vi "SEE_PXI_TopBench_Rev11.vi"() -> ()   [LabVIEW 2019]
uses:
  Controls/DataBlockControl.ctl
  Controls/RFBlockControl.ctl
  <instrlib>/niScope/Controls/niScope vertical coupling.ctl
  Controls/VISA_power_Control.ctl
  Controls/DCPowerBlock_byInstrument_Control.ctl
  Controls/OscilloscopeBlockControl2.ctl
  Controls/PlotColorArray.ctl
panel:
  in  "output cluster":T6 {"Oscilloscope Configuration Input Array"."vertical coupling" items=["AC", "DC", "Ground"]}
  out "DCPowerInformationArrayOutput":T1[](array[typedef])
  in  "DCPowerInformationClusterArray_Input":T1[](array[typedef])
  in  "config file inputs":T7 {"Oscilloscope Configuration Input Array"."vertical coupling" items=["AC", "DC", "Ground"]}
  out "VISAPowerOutputArray":T2[](array[typedef])
  out "OscilloscopeInfoArray":T8(array[cluster]) {"vertical coupling" items=["AC", "DC", "Ground"]}
  out "RFBlockInfoArray":T3[](array[typedef])
  out "error in":errorcluster
  out "Run Parameters":T9
  in  "stop":bool
  out "Configuration Dashboard":bool[](array[boolean])
  in  "Data Collection Block":bool
  in  "Oscilloscope Block":bool
  in  "Power Block":bool
  in  "RF Block":bool
  in  "Data Block":bool
  in  "Reset":bool
  # "Instructions:\nProgress through the configuration dashboard, note the arrays to the right to confirm settings. Once everything is configured, you can begin data collection"
  # "IMPORTANT NOTES\n\nALL LEDs must be lit up before you can begin data collection. Even if you don't need an RF source or oscilloscope, you still just open up the system and then exit (you don't need to configure one.\n\nAfter data collection, you will have the option to reset the system or keep the configuration.\n\nOnly press \"stop\" if you are completely done with collecting data or if the program does not allow you to open another subvi\n\nIf you get a \"running an implicit call\" just restart the program"
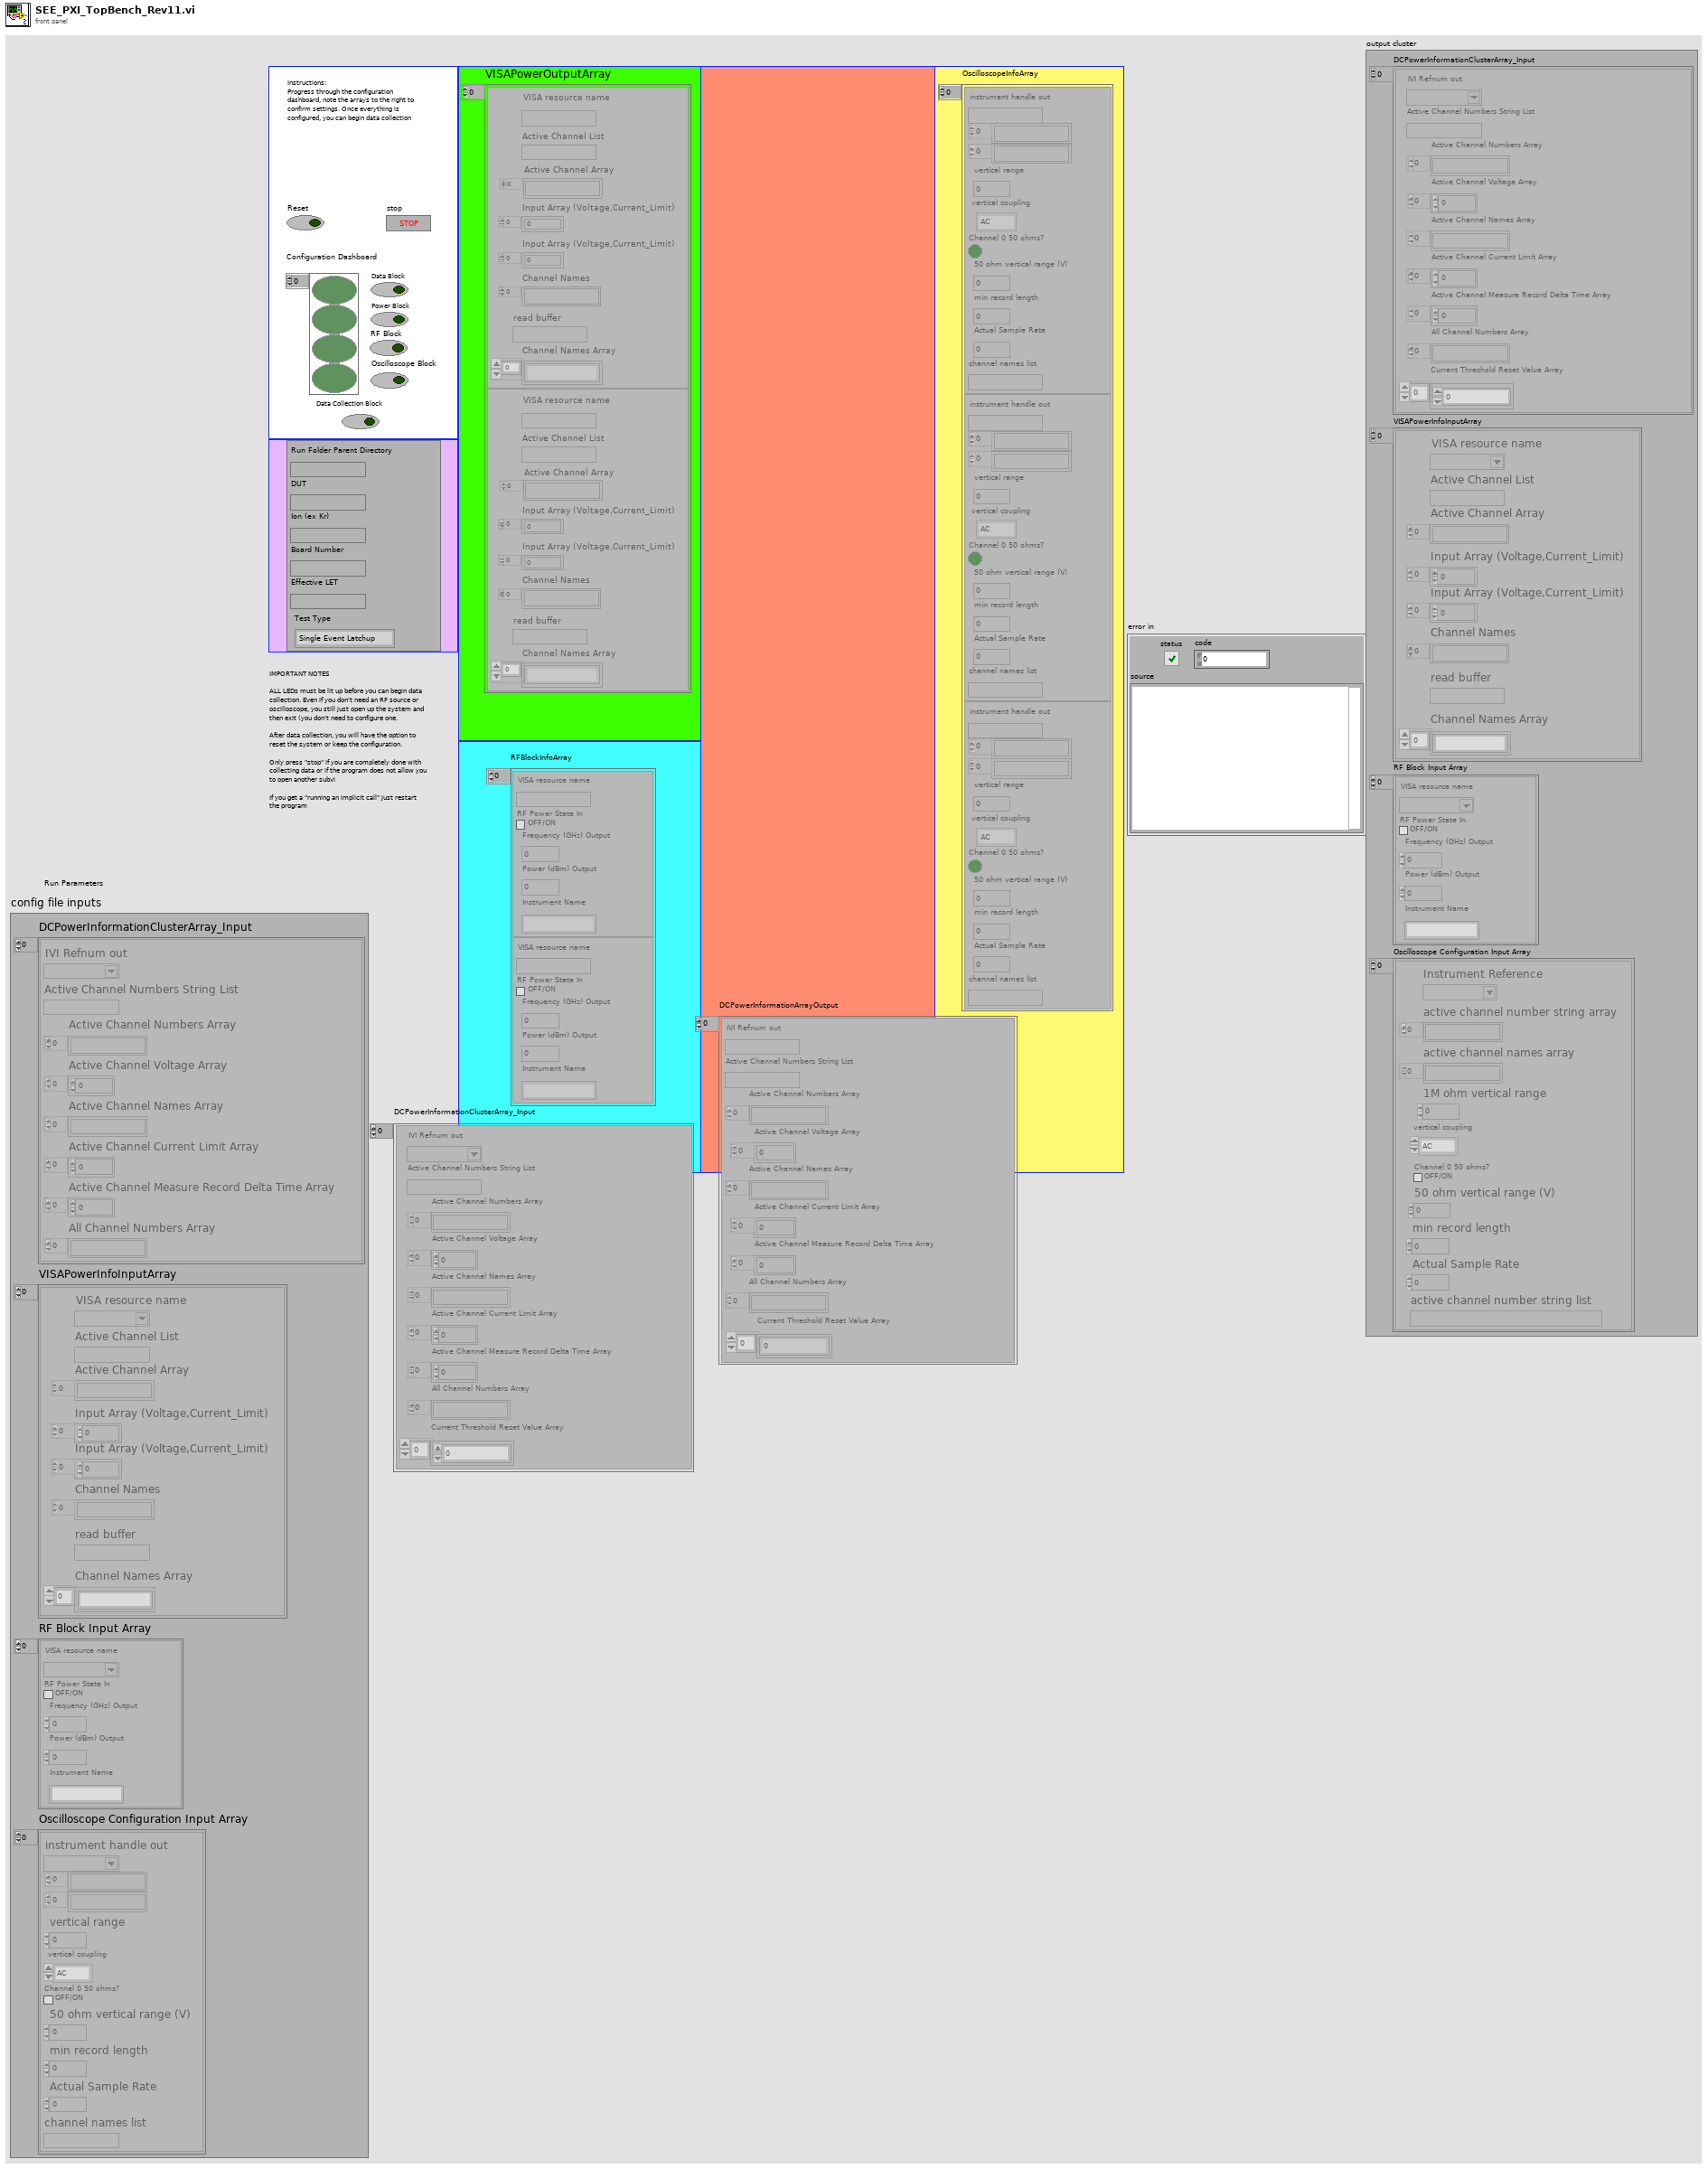
[diagram p1: front panel]
types:
  T1 = typedef "DCPowerBlock_byInstrument_Control.ctl" = cluster{"IVI Refnum out":refnum<k15>, "Active Channel Numbers String List":string, "Active Channel Numbers Array":string[], "Active Channel Voltage Array":dbl[], "Active Channel Names Array":string[], "Active Channel Current Limit Array":dbl[], "Active Channel Measure Record Delta Time Array":dbl[], "All Channel Numbers Array":string[], "Current Threshold Reset Value Array":dbl[]}
  T2 = typedef "VISA_power_Control.ctl" = cluster{"VISA resource name":refnum<visa-resource-name>, "Active Channel List":string, "Active Channel Array":string[], "Input Array (Voltage,Current_Limit)":dbl[], "Input Array (Voltage,Current_Limit)":dbl[], "Channel Names":string[], "read buffer":string, "Channel Names Array":string[]}
  T3 = typedef "RFBlockControl.ctl" = cluster{"VISA resource name":refnum<visa-resource-name>, "RF Power State In":bool, "Frequency (GHz) Output":dbl, "Power (dBm) Output":dbl, "Instrument Name":string}
  T4 = typedef "OscilloscopeBlockControl2.ctl" = cluster{"Instrument Reference":refnum<k15>, "active channel number string array":string[], "active channel names array":string[], "1M ohm vertical range":dbl, "vertical coupling":T5, "Channel 0 50 ohms?":bool, "50 ohm vertical range (V)":dbl, "min record length":i32, "Actual Sample Rate":dbl, "active channel number string list":string}
  T5 = typedef "niScope vertical coupling.ctl" = i32
  T6 = cluster{"DCPowerInformationClusterArray_Input":T1[], "VISAPowerInfoInputArray":T2[], "RF Block Input Array":T3[], "Oscilloscope Configuration Input Array":T4[]}
  T7 = cluster{"DCPowerInformationClusterArray_Input":cluster{"IVI Refnum out":refnum<k15>, "Active Channel Numbers String List":string, "Active Channel Numbers Array":string[], "Active Channel Voltage Array":dbl[], "Active Channel Names Array":string[], "Active Channel Current Limit Array":dbl[], "Active Channel Measure Record Delta Time Array":dbl[], "All Channel Numbers Array":string[]}[], "VISAPowerInfoInputArray":T2[], "RF Block Input Array":T3[], "Oscilloscope Configuration Input Array":cluster{"instrument handle out":refnum<k15>, string[], string[], "vertical range":dbl, "vertical coupling":T5, "Channel 0 50 ohms?":bool, "50 ohm vertical range (V)":dbl, "min record length":i32, "Actual Sample Rate":dbl, "channel names list":string}[]}
  T8 = cluster{"instrument handle out":refnum<k15>, string[], string[], "vertical range":dbl, "vertical coupling":T5, "Channel 0 50 ohms?":bool, "50 ohm vertical range (V)":dbl, "min record length":i32, "Actual Sample Rate":dbl, "channel names list":string}[]
  T9 = typedef "DataBlockControl.ctl" = cluster{"Run Folder Parent Directory":path, "DUT":string, "Ion (ex Kr)":string, "Board Number":string, "Effective LET":string, "Test Type":enum16{"Single Event Latchup", "Single Event Transient", "Single Event Upset"}}
  T10 = cluster{"product_name":string, "register_read_array":dbl[], "performance_check":string, "campaign":string, "logic_path":string, "logic_name":string, "power_supplies":cluster{"Supply_Number":dbl, "Supply_Array":cluster{"instr_name":string, "voltage":dbl, "supply_name":string, "channel":string, "current_limit":dbl, "measure_record_length":dbl, "aperature_time":dbl}[]}, "signal_generators":cluster{"Gen_Number":dbl, "Gen_Array":cluster{"GPIB_address":dbl, "signal_name":string, "frequency":dbl, "power":dbl}[]}, "expected_register_values":cluster{"Reg_0x3":string}}
  T11 = typedef "PlotColorArray.ctl" = u32[]
  T12 = cluster{"instrument handle out":refnum<k15>, string, string[], dbl[], string[], "Current Limit Output Array":dbl[], dbl[]}[]
  T13 = cluster{"DCPowerInformationClusterArray_Input":cluster{"IVI Refnum out":refnum<k15>, "Active Channel Numbers String List":string, "Active Channel Numbers Array":string[], "Active Channel Voltage Array":dbl[], "Active Channel Names Array":string[], "Active Channel Current Limit Array":dbl[], "Active Channel Measure Record Delta Time Array":dbl[], "All Channel Numbers Array":string[]}[], "VISAPowerInfoInputArray":cluster{"VISA resource name":refnum<visa-resource-name>, "String List":string, string[], "Input Array (Voltage,Current_Limit)":dbl[], "Input Array (Voltage,Current_Limit)":dbl[], "Channel Names":string[], "read buffer":string}[], "RF Block Input Array":T3[], "Oscilloscope Configuration Input Array":cluster{"instrument handle out":refnum<k15>, string[], string[], "vertical range":dbl, "vertical coupling":T5, "Channel 0 50 ohms?":bool, "50 ohm vertical range (V)":dbl, "min record length":i32, "Actual Sample Rate":dbl, "channel names list":string}[]}
  T14 = cluster{"VISA resource name":refnum<visa-resource-name>, "String List":string, string[], "Input Array (Voltage,Current_Limit)":dbl[], "Input Array (Voltage,Current_Limit)":dbl[], "Channel Names":string[], "read buffer":string}[]
  T15 = cluster{"IVI Refnum out":refnum<k15>, "Active Channel Numbers String List":string, "Active Channel Numbers Array":string[], "Active Channel Voltage Array":dbl[], "Active Channel Names Array":string[], "Active Channel Current Limit Array":dbl[], "Active Channel Measure Record Delta Time Array":dbl[], "All Channel Numbers Array":string[]}[]
  T16 = cluster{"IVI Refnum out":refnum<k15>, "String List":string, string[], dbl[], string[], dbl[], dbl[], string[], dbl[]}[]
  T17 = cluster{"instrument handle out":refnum<k15>, "channel numbers array":string[], "channel names array":string[], "vertical range":dbl, "vertical coupling":T5, "Channel 0 50 ohms?":bool, "50 ohm vertical range (V)":dbl, "min record length":i32, "Actual Sample Rate":dbl}[]
  T18 = enum16{"Single Event Latchup", "Single Event Transient", "Single Event Upset"}
  T19 = cluster{"Array of fetched data":dbl[][], string, i32[]}[]
  T20 = cluster{"Array of fetched data":dbl[][], string, i32[]}[][]
  T21 = cluster{"Array of fetched data":dbl[][], string, i32[]}
  T22 = cluster{"IVI Refnum out":refnum<k15>, "Active Channel Numbers String List":string, "Active Channel Numbers Array":string[], "Active Channel Voltage Array":dbl[], "Active Channel Names Array":string[], "Active Channel Current Limit Array":dbl[], "Active Channel Measure Record Delta Time Array":dbl[], "All Channel Numbers Array":string[], dbl[]}[]
  T23 = cluster{"DCPowerInformationClusterArray_Input out":cluster{"IVI Refnum out":refnum<k15>, "Active Channel Numbers String List":string, "Active Channel Numbers Array":string[], "Active Channel Voltage Array":dbl[], "Active Channel Names Array":string[], "Active Channel Current Limit Array":dbl[], "Active Channel Measure Record Delta Time Array":dbl[], "All Channel Numbers Array":string[]}[], "VISAPowerInfoInputArray":cluster{"VISA resource name":refnum<visa-resource-name>, "String List":string, string[], "Input Array (Voltage,Current_Limit)":dbl[], "Input Array (Voltage,Current_Limit)":dbl[], "Channel Names":string[], "read buffer":string}[], "RF Block Input Array out":T3[], "Oscilloscope Configuration Input Array":cluster{"instrument handle out":refnum<k15>, string[], string[], "vertical range":dbl, "vertical coupling":T5, "Channel 0 50 ohms?":bool, "50 ohm vertical range (V)":dbl, "min record length":i32, "Actual Sample Rate":dbl, "channel names list":string}[]}
  T24 = cluster{"path out":path, string, "Ion (ex Kr)":string, "Board Number":string, "Effective LET":string, "Test Type":enum16{"Single Event Latchup", "Single Event Transient", "Single Event Upset"}}
  T25 = cluster{"DCPowerInformationClusterArray out":T1[], "VISAPowerInfoOutputArray":T2[], "RF Block Input Array out":T3[], "Oscilloscope Configuration Input Array":T4[]}
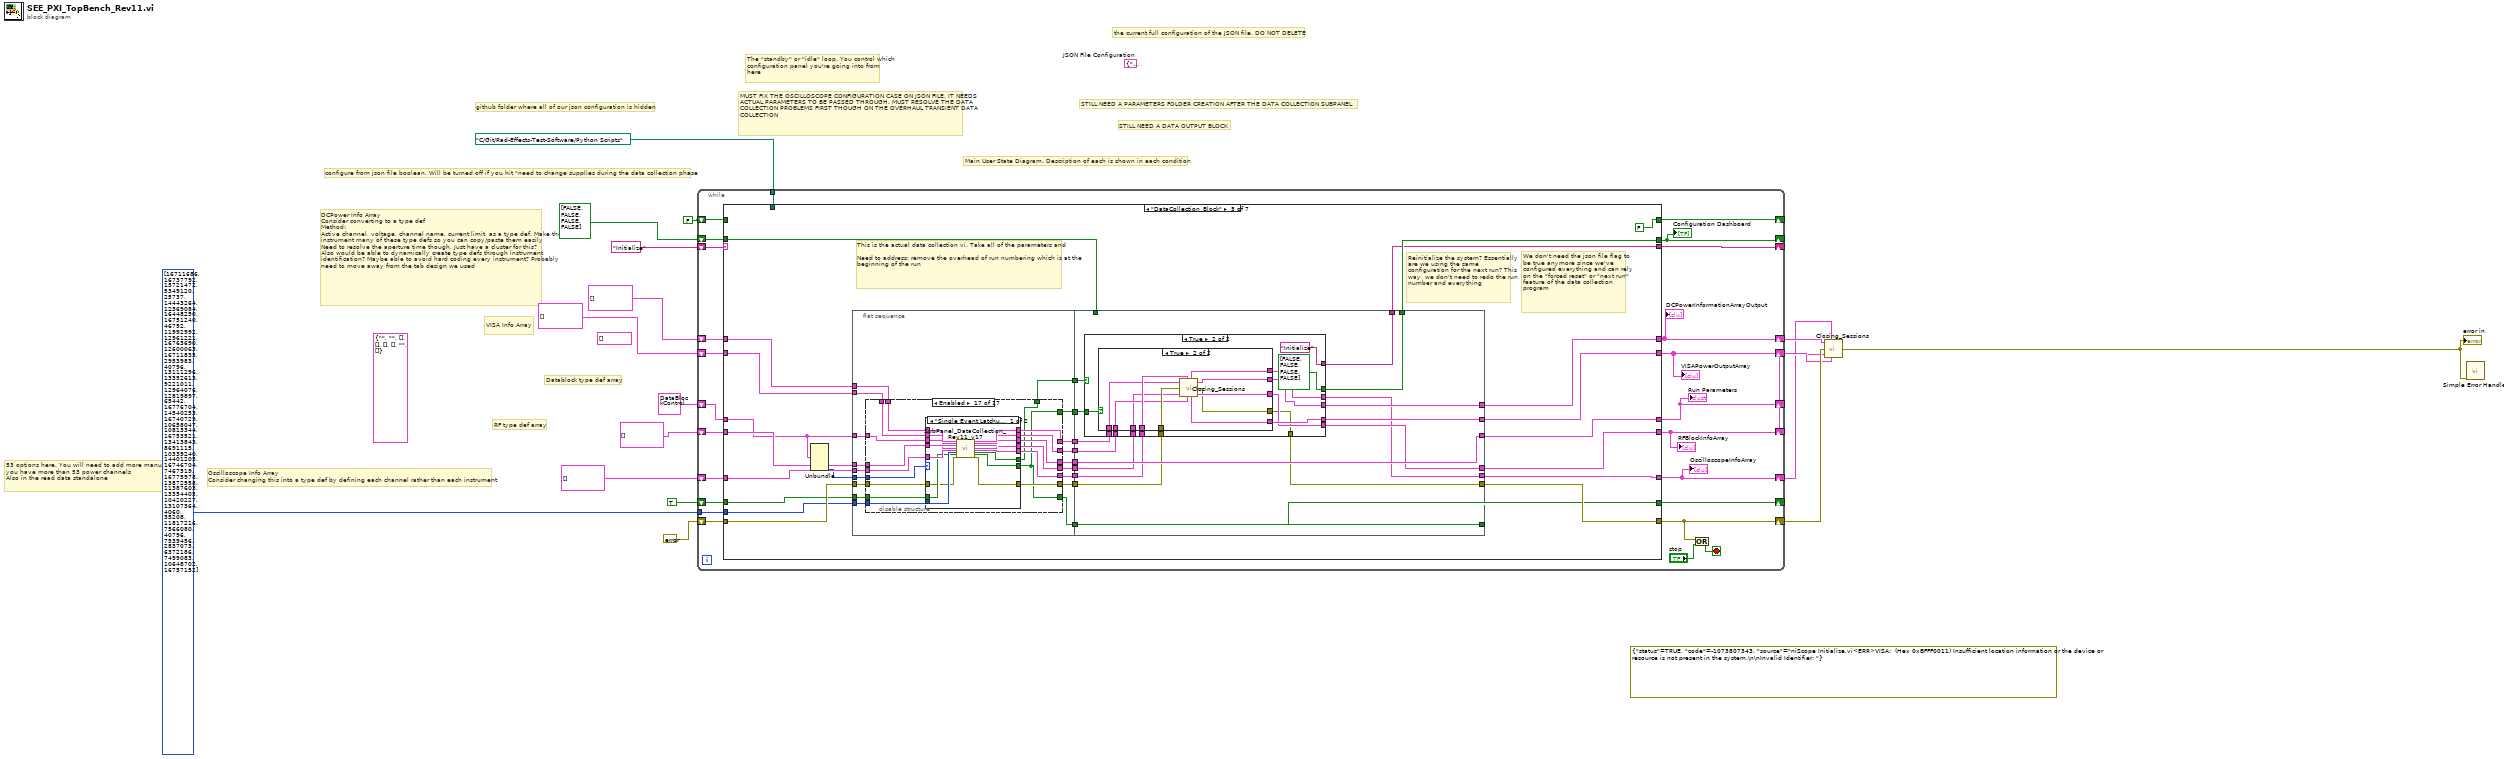
[diagram p0: block diagram]
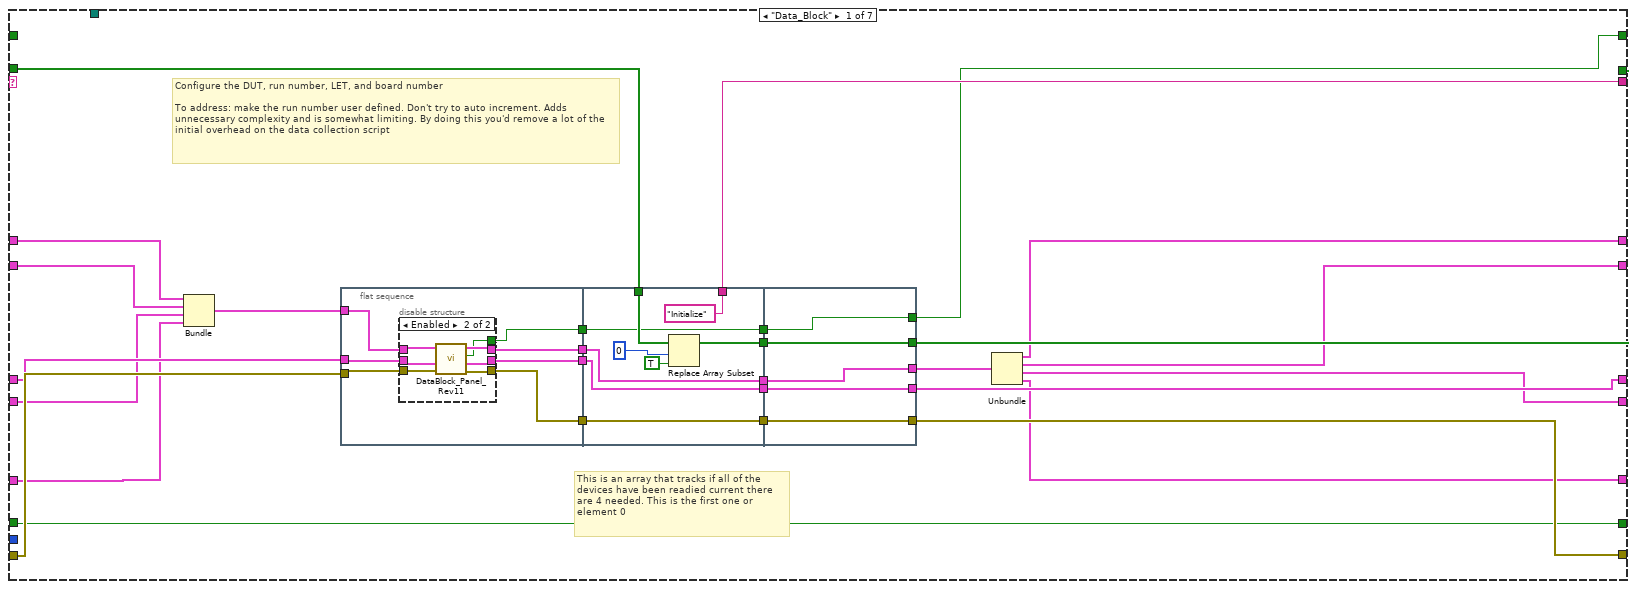
[diagram p2: hidden frame]
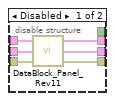
[diagram p3: hidden frame]
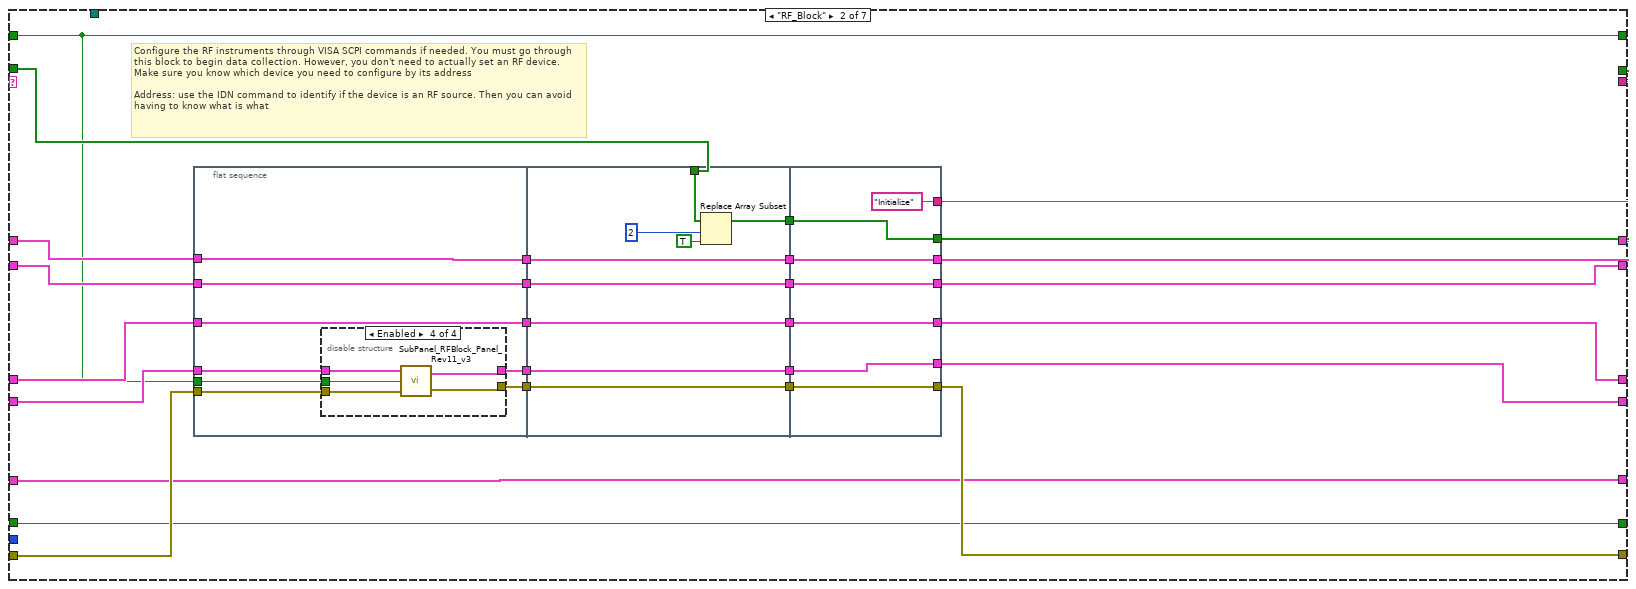
[diagram p4: hidden frame]
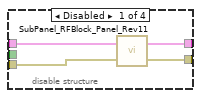
[diagram p5: hidden frame]
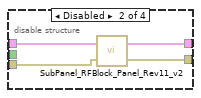
[diagram p6: hidden frame]
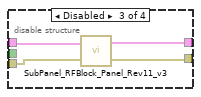
[diagram p7: hidden frame]
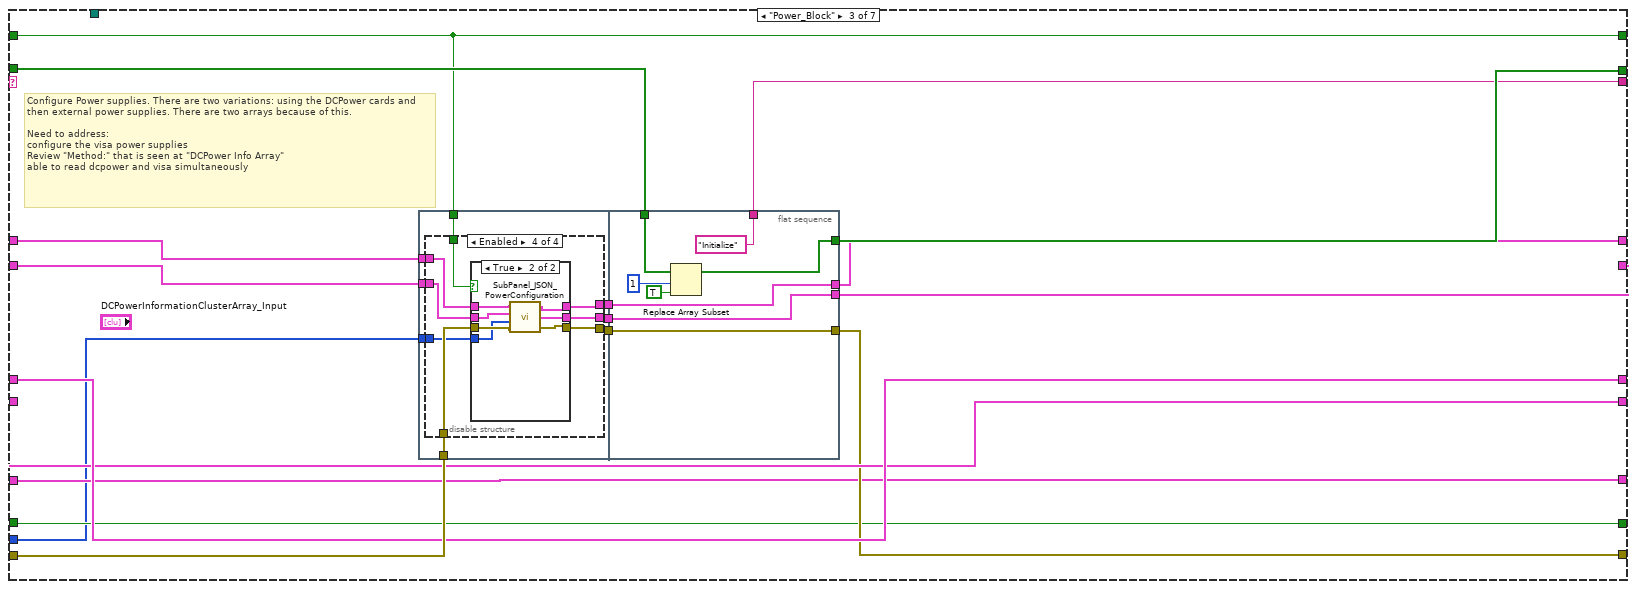
[diagram p8: hidden frame]
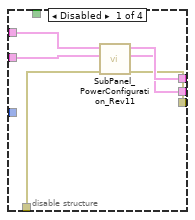
[diagram p9: hidden frame]
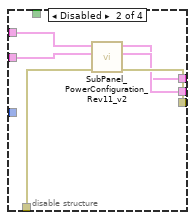
[diagram p10: hidden frame]
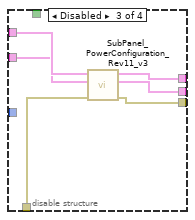
[diagram p11: hidden frame]
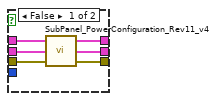
[diagram p12: hidden frame]
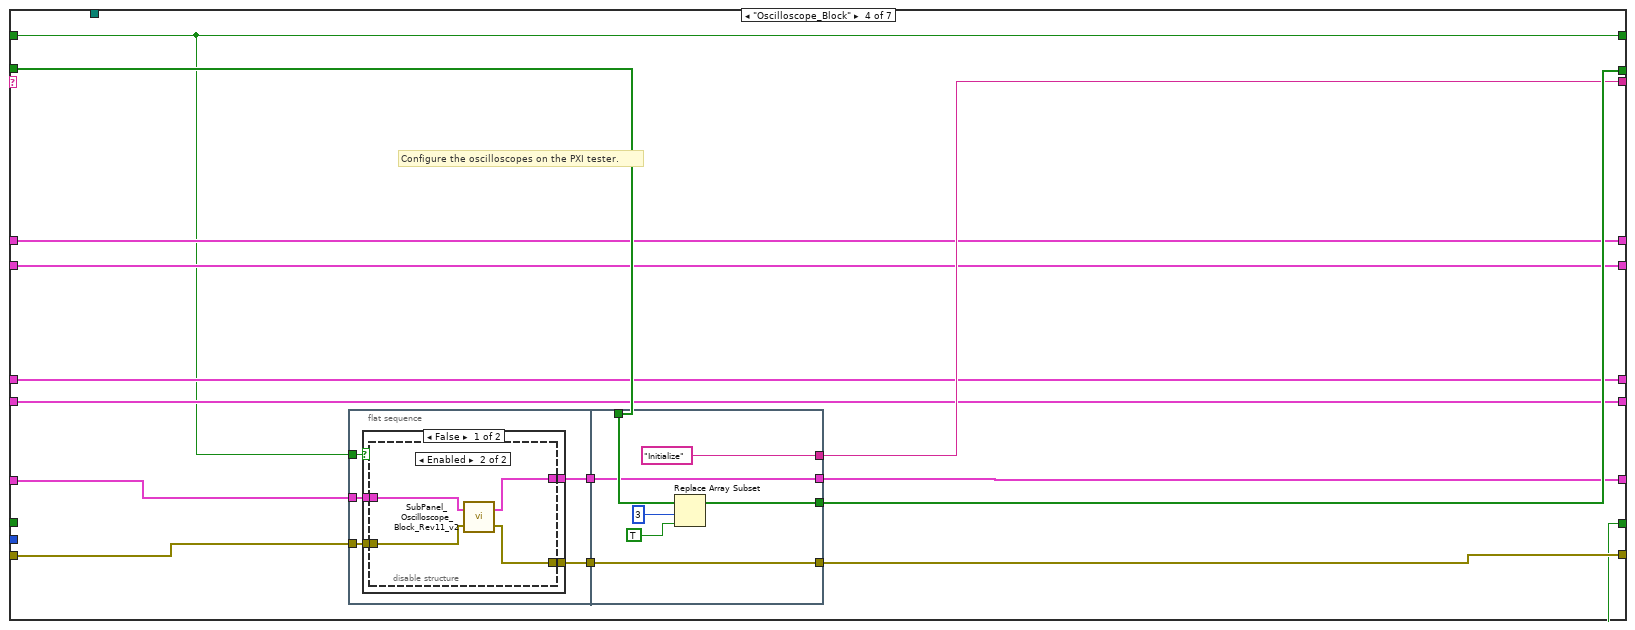
[diagram p13: hidden frame]
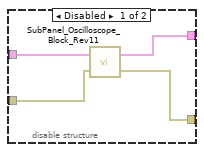
[diagram p14: hidden frame]
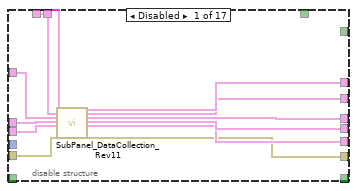
[diagram p16: hidden frame]
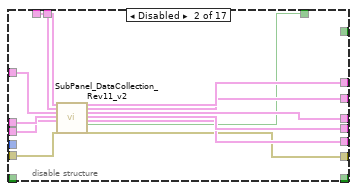
[diagram p17: hidden frame]
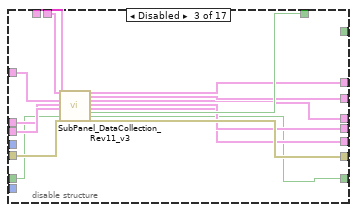
[diagram p18: hidden frame]
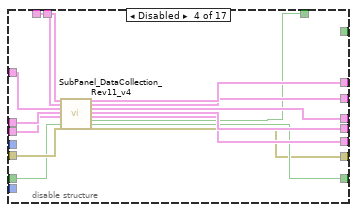
[diagram p19: hidden frame]
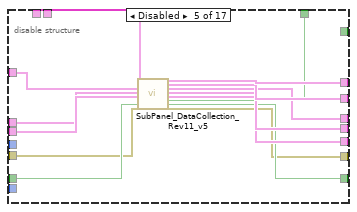
[diagram p20: hidden frame]
diagram:
  (unwired) errorcluster {"status"=TRUE, "code"=-1073807343, "source"="niScope Initialize.vi<ERR>VISA:  (Hex 0xBFFF0011) Insufficient location information or the device or resource is not present in the system.\n\nInvalid Identifier: "} ("error out")
  (unwired) T2 {"VISA resource name"="", "Active Channel List"="", "Active Channel Array"=[], "Input Array (Voltage,Current_Limit)"=[], "Input Array (Voltage,Current_Limit)"=[], "Channel Names"=[], "read buffer"="", "Channel Names Array"=[]}
  (unwired) T10 {"product_name"="", "register_read_array"=[], "performance_check"="", "campaign"="", "logic_path"="", "logic_name"="", "power_supplies"={"Supply_Number"=0.0, "Supply_Array"=[]}, "signal_generators"={"Gen_Number"=0.0, "Gen_Array"=[]}, "expected_register_values"={"Reg_0x3"=""}}  # JSON File Configuration
  (unwired) T12 [] ("DCPowerInformationClusterArray_Input")
  # "the current full configuration of the JSON file. DO NOT DELETE"
  # "github folder where all of our json configuration is hidden"
  # "MUST FIX THE OSCILLOSCOPE CONFIGURATION CASE ON JSON FILE. IT NEEDS ACTUAL PARAMETERS TO BE PASSED THROUGH. MUST RESOLVE THE DATA COLLECTION PROBLEMS FIRST THOUGH ON THE OVERHAUL TRANSIENT DATA COLLECTION"
  # "The \"standby\" or \"idle\" loop. You control which configuration panel you're going into from here"
  # "configure from json file boolean. Will be turned off if you hit \"need to change supplies during the data collection phase"
  # "DCPower Info Array\nConsider converting to a type def\nMethod:\nActive channel, voltage, channel name, current limit, as a type def. Make the instrument many of these type defs so you can copy/paste them easily\nNeed to resolve the aperture time though. Just have a cluster for this?\nAlso would be able to dynamically create type defs through instrument identification? Maybe able to avoid hard coding every instrument? Probably need to move away from the tab design we used"
  # "Datablock type def array"
  # "RF type def array"
  # "Main User State Diagram. Description of each is shown in each condition"
  # "53 options here. You will need to add more manually if you have more than 53 power channels\nAlso in the read data standalone"
  # "STILL NEED A DATA OUTPUT BLOCK"
  # "STILL NEED A PARAMETERS FOLDER CREATION AFTER THE DATA COLLECTION SUBPANEL"
  # "Oscilloscope Info Array\nConsider changing this into a type def by defining each channel rather than each instrument"
  # "VISA Info Array"
  n1 = while {
    shift-right: [w40] -> _
    shift-left: bool[] [FALSE, FALSE, FALSE, FALSE] -> [w41]
    shift-right: [w39] -> _
    shift-left: "Initialize" -> [w42]
    shift-right: [w20] -> w12
    shift-left: errorcluster {"status"=FALSE, "code"=0, "source"=""} ("error in") -> [w38]
    shift-right: [w36] -> _
    shift-left: T9 {"Run Folder Parent Directory"=path "", "DUT"="", "Ion (ex Kr)"="", "Board Number"="", "Effective LET"="", "Test Type"=enum."Single Event Latchup"} ("Run Data SubPanel Input") -> [w37]
    shift-right: [w34] -> w10
    shift-left: T3[] [] ("RF Block Input Array") -> [w35]
    shift-right: [w30] -> w13
    shift-left: T1[] [] ("DCPowerInformationClusterArray_Input") -> [w33]
    shift-right: [w31] -> w11
    shift-left: T2[] [] ("VISAPowerInfoInputArray") -> [w32]
    shift-right: [w28] -> w7
    shift-left: T4[] [] ("Oscilloscope Configuration Input Array") -> [w29]
    shift-right: [w26] -> _
    shift-left: TRUE ("New Run?") -> [w27]
    tunnel: T11 [16711686, 16737792, 15721472, 5349120, 25737, 14443264, 12369084, 16448250, 16751240, 46792, 11992992, 12961221, 16763690, 12600063, 16711835, 2953983, 40796, 13111296, 13352613, 9221011, 12964076, 12819897, 65442, 16776704, 14540253, 16740729, 10658047, 10813344, 16753521, 13413843, 8691115, 10339240, 14401205, 16746704, 7467519, 16775978, 13872558, 11387603, 13354405, 10420227, 13107364, 4060, 35208, 11817216, 7566080, 40796, 7539456, 2837073, 6372186, 7499083, 10648702, 16757152] ("Array") -> [w25]
    shift-right: [w24] -> _
    shift-left: FALSE ("Configuring From JSON file?") -> [w23]
    tunnel: path "C:/Git/Rad-Effects-Test-Software/Python Scripts" ("file path (use dialog)") -> [w19]
    stop <- w21 stop-if-true
    n2 = case shown="\"DataCollection_Block\"" w42 {
      selector: w42 -> [_ _ _ _ _ w685 _]
      tunnel: w41 -> [w70 w128 w186 w260 w299 w676 w786]
      tunnel: [w69 w127 w185 w259 w298 w686 w785] -> w40
      tunnel: [w67 w131 w184 w258 w297 w684 w788] -> w39
      tunnel: w38 -> [w66 w130 w189 w253 w311 w683 w792]
      tunnel: [w65 w129 w178 w252 w301 w683 w791] -> w20
      tunnel: w37 -> [w62 w117 w188 w255 w290 w682 w784]
      tunnel: [w61 w116 w188 w255 w306 w682 w783] -> w36
      tunnel: w35 -> [w57 w123 w187 w254 w313 w681 w798]
      tunnel: [w47 w122 w187 w254 w304 w681 w795] -> w34
      tunnel: w33 -> [w56 w112 w190 w257 w315 w680 w800]
      tunnel: w32 -> [w55 w108 w173 w256 w314 w679 w799]
      tunnel: [w49 w115 w183 w257 w310 w680 w793] -> w30
      tunnel: [w48 w111 w181 w256 w308 w679 w794] -> w31
      tunnel: w29 -> [w50 w107 w177 w250 w312 w678 w797]
      tunnel: [w46 w107 w177 w249 w291 w678 w796] -> w28
      tunnel: w27 -> [w58 w106 w176 w247 w295 w677 w802]
      tunnel: [w58 w106 w176 w247 w293 w677 w802] -> w26
      tunnel: w25 -> [_ _ w174 _ w292 _ _]
      tunnel: [w45 w105 w175 w246 FALSE ("Configuring From JSON file?") w675 w787] -> w24
      tunnel: w23 -> [_ w105 w175 w246 _ w675 _]
      tunnel: w19 -> [_ _ _ _ _ _ w789]
      frame "Data_Block" {
        # "This is an array that tracks if all of the devices have been readied current there are 4 needed. This is the first one or element 0"
        # "Configure the DUT, run number, LET, and board number\n\nTo address: make the run number user defined. Don't try to auto increment. Adds unnecessary complexity and is somewhat limiting. By doing this you'd remove a lot of the initial overhead on the data collection script"
        n3 = Bundle("DCPowerInformationClusterArray_Input"=w56, "VISAPowerInfoInputArray"=w55, "RF Block Input Array"=w57, "Oscilloscope Configuration Input Array"=w50) -> (w54:T6)  [unwired: 1 in]
        n4 = flat-sequence {
          tunnel: w66 -> [w77]
          tunnel: [w76] -> w63
          tunnel: w62 -> [w74]
          tunnel: [w75] -> w59
          tunnel: w54 -> [w72]
          tunnel: [w73] -> w52
          tunnel: [w71] -> w43
          tunnel: w70 -> [w99]
          tunnel: [w96] -> w68
          tunnel: ["Initialize"] -> w67
          tunnel: [w94] -> w64
          tunnel: w63 -> [w94]
          tunnel: [w93] -> w60
          tunnel: w59 -> [w93]
          tunnel: [w92] -> w53
          tunnel: w52 -> [w92]
          tunnel: [w91] -> w44
          tunnel: w43 -> [w91]
          tunnel: [w104] -> w69
          tunnel: w68 -> [w104]
          tunnel: [w103] -> w65
          tunnel: w64 -> [w103]
          tunnel: [w102] -> w61
          tunnel: w60 -> [w102]
          tunnel: [w101] -> w51
          tunnel: w53 -> [w101]
          tunnel: [w100] -> w45
          tunnel: w44 -> [w100]
          frame #0 {
            n5 = disable-structure shown="Enabled" {
              disable-tunnel: w77 -> [w83 w89]
              disable-tunnel: [w82 w86] -> w76
              disable-tunnel: [w81 w85] -> w75
              disable-tunnel: w74 -> [w80 w90]
              disable-tunnel: [w79 w87] -> w73
              disable-tunnel: w72 -> [w78 w88]
              disable-tunnel: [_ w84] -> w71
              frame Disabled {
                n6 = call "DataBlock_Panel_Rev11.vi"("error in"=w83, "Run Data SubPanel Input"=w80, "config file inputs"=w78) -> ("error out"=w82:errorcluster, "Run Data SubPanel Output"=w81:T9, "config file outputs"=w79:T13)
              }
              frame Enabled {
                n7 = call "DataBlock_Panel_Rev11.vi"("error in"=w89, "Run Data SubPanel Input"=w90, "config file inputs"=w88) -> ("error out"=w86:errorcluster, "Run Data SubPanel Output"=w85:T9, "Configuring From JSON file?"=w84:bool, "config file outputs"=w87:T6)  [unwired: 1 in]
              }
            }
          }
          frame #1 {
            n8 = Replace Array Subset(array=w99, new element=TRUE ("new element/subarray"), index=0) -> (w96:bool[])
          }
          frame #2 {
          }
        }
        n9 = Unbundle(w51) -> ("DCPowerInformationClusterArray_Input"=w49:T1[], "VISAPowerInfoInputArray"=w48:T2[], "RF Block Input Array"=w47:T3[], "Oscilloscope Configuration Input Array"=w46:T4[])
      }
      frame "RF_Block" {
        # "Configure the RF instruments through VISA SCPI commands if needed. You must go through this block to begin data collection. However, you don't need to actually set an RF device. Make sure you know which device you need to configure by its address\n\nAddress: use the IDN command to identify if the device is an RF source. Then you can avoid having to know what is what"
        n10 = flat-sequence {
          tunnel: w130 -> [w139]
          tunnel: [w138] -> w124
          tunnel: w123 -> [w137]
          tunnel: [w136] -> w120
          tunnel: [w135] -> w118
          tunnel: w117 -> [w135]
          tunnel: [w134] -> w113
          tunnel: w112 -> [w134]
          tunnel: [w133] -> w109
          tunnel: w108 -> [w133]
          tunnel: w105 -> [w132]
          tunnel: w128 -> [w165]
          tunnel: [w162] -> w126
          tunnel: [w161] -> w125
          tunnel: w124 -> [w161]
          tunnel: [w160] -> w121
          tunnel: w120 -> [w160]
          tunnel: [w159] -> w119
          tunnel: w118 -> [w159]
          tunnel: [w158] -> w114
          tunnel: w113 -> [w158]
          tunnel: [w157] -> w110
          tunnel: w109 -> [w157]
          tunnel: ["Initialize"] -> w131
          tunnel: [w170] -> w129
          tunnel: [w171] -> w127
          tunnel: w126 -> [w171]
          tunnel: w125 -> [w170]
          tunnel: [w169] -> w122
          tunnel: w121 -> [w169]
          tunnel: [w168] -> w116
          tunnel: w119 -> [w168]
          tunnel: [w167] -> w115
          tunnel: w114 -> [w167]
          tunnel: [w166] -> w111
          tunnel: w110 -> [w166]
          frame #0 {
            n11 = disable-structure shown="Enabled" {
              disable-tunnel: w139 -> [w143 w146 w150 w155]
              disable-tunnel: [w142 w144 w149 w152] -> w138
              disable-tunnel: w137 -> [w141 w147 w151 w156]
              disable-tunnel: [w140 w145 w148 w153] -> w136
              disable-tunnel: w132 -> [_ _ _ w154]
              frame Disabled {
                n12 = call "SubPanel_RFBlock_Panel_Rev11.vi"("error input"=w143, "RF Block Input"=w141) -> ("error output"=w142:errorcluster, "RF Block Output"=w140:T3)
              }
              frame Disabled {
                n13 = call "SubPanel_RFBlock_Panel_Rev11_v2.vi"("error input"=w146, "RF Block Input Array"=w147) -> ("error output"=w144:errorcluster, "RF Block Output Array"=w145:T3[])
              }
              frame Disabled {
                n14 = call "SubPanel_RFBlock_Panel_Rev11_v3.vi"("error input"=w150, "RF Block Input Array"=w151) -> ("error output"=w149:errorcluster, "RF Block Output Array"=w148:T3[])
              }
              frame Enabled {
                n15 = call "SubPanel_RFBlock_Panel_Rev11_v3.vi"("error input"=w155, "JSON file configuration?"=w154, "RF Block Input Array"=w156) -> ("error output"=w152:errorcluster, "RF Block Output Array"=w153:T3[])
              }
            }
          }
          frame #1 {
            n16 = Replace Array Subset(array=w165, new element=TRUE ("new element/subarray"), index=2) -> (w162:bool[])
          }
          frame #2 {
          }
        }
      }
      frame "Power_Block" {
        # "Configure Power supplies. There are two variations: using the DCPower cards and then external power supplies. There are two arrays because of this.  \n\nNeed to address:\nconfigure the visa power supplies\nReview \"Method:\" that is seen at \"DCPower Info Array\"\nable to read dcpower and visa simultaneously"
        n17 = flat-sequence {
          tunnel: w190 -> [w198]
          tunnel: w173 -> [w197]
          tunnel: w189 -> [w196]
          tunnel: [w195] -> w182
          tunnel: [w194] -> w180
          tunnel: [w193] -> w179
          tunnel: w175 -> [w192]
          tunnel: w174 -> [w191]
          tunnel: w186 -> [w243]
          tunnel: [w242] -> w185
          tunnel: ["Initialize"] -> w184
          tunnel: [w240] -> w183
          tunnel: w182 -> [w240]
          tunnel: [w239] -> w181
          tunnel: w180 -> [w239]
          tunnel: [w238] -> w178
          tunnel: w179 -> [w238]
          frame #0 {
            n18 = disable-structure shown="Enabled" {
              disable-tunnel: w198 -> [w204 w205 w213 w219]
              disable-tunnel: w197 -> [w203 w206 w212 w220]
              disable-tunnel: w196 -> [w202 w210 w211 w221]
              disable-tunnel: [w201 w207 w214 w224] -> w195
              disable-tunnel: [w200 w208 w215 w223] -> w194
              disable-tunnel: [w199 w209 w216 w222] -> w193
              disable-tunnel: w192 -> [_ _ _ w217]
              disable-tunnel: w191 -> [_ _ _ w218]
              frame Disabled {
                n19 = call "SubPanel_PowerConfiguration_Rev11.vi"("error in"=w202, "VISAPowerInfoInputArray"=w203, "DCPowerInformationClusterArray_Input"=w204) -> ("error out"=w199:errorcluster, "VISAPowerInfoOutputArray"=w200:T14, "DCPowerInformationClusterArray_Output"=w201:T12)  [unwired: 6 in]
              }
              frame Disabled {
                n20 = call "SubPanel_PowerConfiguration_Rev11_v2.vi"("error in"=w210, "VISAPowerInfoInputArray"=w206, "DCPowerInformationClusterArray_Input"=w205) -> ("error out"=w209:errorcluster, "VISAPowerInfoOutputArray"=w208:T14, "DCPowerInformationClusterArray_Output"=w207:T15)  [unwired: 6 in]
              }
              frame Disabled {
                n21 = call "SubPanel_PowerConfiguration_Rev11_v3.vi"("error in"=w211, "VISAPowerInfoInputArray"=w212, "DCPowerInformationClusterArray_Input"=w213) -> ("error out"=w216:errorcluster, "VISAPowerInfoOutputArray"=w215:T14, "DCPowerInformationClusterArray_Output"=w214:T15)  [unwired: 6 in]
              }
              frame Enabled {
                n22 = case shown="True" w217 {
                  tunnel: [w230 w234] -> w224
                  tunnel: [w229 w232] -> w223
                  tunnel: [w228 w233] -> w222
                  tunnel: w221 -> [w227 w236]
                  tunnel: w220 -> [w226 w231]
                  tunnel: w219 -> [w225 w237]
                  tunnel: w218 -> [_ w235]
                  frame False {
                    n23 = call "SubPanel_PowerConfiguration_Rev11_v4.vi"("error in"=w227, "VISAPowerInfoInputArray"=w226, "DCPowerInformationClusterArray_Input"=w225) -> ("error out"=w228:errorcluster, "VISAPowerInfoOutputArray"=w229:T2[], "DCPowerInformationClusterArray_Output"=w230:T1[])
                  }
                  frame True {
                    n24 = call "SubPanel_JSON_PowerConfiguration.vi"("error_input"=w236, "ColorPalette"=w235, "VISAPowerInfoInputArray"=w231, "DCPowerInformationClusterArray_Input"=w237) -> ("error output"=w233:errorcluster, "VISAPowerInfoOutputArray"=w232:T2[], "DCPowerInformation_byInstrument"=w234:T16)
                  }
                }
              }
            }
          }
          frame #1 {
            n25 = Replace Array Subset(array=w243, new element=TRUE ("new element/subarray"), index=1) -> (w242:bool[])
          }
        }
      }
      frame "Oscilloscope_Block" {
        # "Configure the oscilloscopes on the PXI tester."
        n26 = flat-sequence {
          tunnel: w253 -> [w265]
          tunnel: [w264] -> w251
          tunnel: w250 -> [w263]
          tunnel: [w262] -> w248
          tunnel: w246 -> [w261]
          tunnel: w260 -> [w286]
          tunnel: [w283] -> w259
          tunnel: ["Initialize"] -> w258
          tunnel: [w281] -> w252
          tunnel: w251 -> [w281]
          tunnel: [w280] -> w249
          tunnel: w248 -> [w280]
          frame #0 {
            n27 = case shown="False" w261 {
              tunnel: w265 -> [w269 w278]
              tunnel: [w268 w278] -> w264
              tunnel: w263 -> [w267 w279]
              tunnel: [w266 w279] -> w262
              frame False {
                n28 = disable-structure shown="Enabled" {
                  disable-tunnel: w269 -> [w273 w275]
                  disable-tunnel: [w272 w274] -> w268
                  disable-tunnel: w267 -> [w271 w277]
                  disable-tunnel: [w270 w276] -> w266
                  frame Disabled {
                    n29 = call "SubPanel_Oscilloscope_Block_Rev11.vi"("error input"=w273, "Oscilloscope Configuration Input Array"=w271) -> ("error out"=w272:errorcluster, "Oscilloscope Configuration Output Array"=w270:T17)
                  }
                  frame Enabled {
                    n30 = call "SubPanel_Oscilloscope_Block_Rev11_v2.vi"("error input"=w275, "Oscilloscope Configuration Input Array"=w277) -> ("error out"=w274:errorcluster, "Oscilloscope Configuration Output Array"=w276:T8)
                  }
                }
              }
              frame True {
              }
            }
          }
          frame #1 {
            n31 = Replace Array Subset(array=w286, new element=TRUE ("new element/subarray"), index=3) -> (w283:bool[])
          }
        }
      }
      frame "DataCollection_Block" {
        # "We don't need the json file flag to be true anymore since we've configured everything and can rely on the \"forced reset\" or \"next run\" feature of the data collection program"
        # "Reinitialize the system? Essentially are we using the same configuration for the next run? This way, we don't need to redo the run number and everything"
        # "This is the actual data collection vi. Take all of the parameters and \n\nNeed to address: remove the overhead of run numbering which is at the beginning of the run"
        n32 = Unbundle(w290) -> ("Test Type"=w289:T18)  [unwired: 5 out]
        n33 = flat-sequence {
          tunnel: w315 -> [w333]
          tunnel: w314 -> [w332]
          tunnel: w290 -> [w331]
          tunnel: w313 -> [w330]
          tunnel: w312 -> [w329]
          tunnel: w311 -> [w328]
          tunnel: [w327] -> w309
          tunnel: [w326] -> w307
          tunnel: [w325] -> w305
          tunnel: [w324] -> w303
          tunnel: [w323] -> w302
          tunnel: [w322] -> w300
          tunnel: [w321] -> w296
          tunnel: w295 -> [w320]
          tunnel: [w319] -> w294
          tunnel: w292 -> [w318]
          tunnel: w289 -> [w317]
          tunnel: [w316] -> w287
          tunnel: [w631] -> w310
          tunnel: w309 -> [w632]
          tunnel: [w630] -> w308
          tunnel: w307 -> [w633]
          tunnel: [w639] -> w306
          tunnel: w305 -> [w639]
          tunnel: [w629] -> w304
          tunnel: w303 -> [w628]
          tunnel: [w626] -> w291
          tunnel: w302 -> [w627]
          tunnel: [w624] -> w301
          tunnel: w300 -> [w625]
          tunnel: w299 -> [_]
          tunnel: [w638] -> w298
          tunnel: [w637] -> w297
          tunnel: w296 -> [w636]
          tunnel: [w635] -> w293
          tunnel: w294 -> [w635]
          tunnel: w287 -> [w634]
          frame #0 {
            n34 = disable-structure shown="Enabled" {
              disable-tunnel: w333 -> [w345 w351 w367 w393 w398 w427 w428 w449 w466 w487 w494 w517 w533 w541 w558 w581 w598]
              disable-tunnel: w332 -> [w344 w350 w368 w392 w399 w426 w429 w448 w467 w486 w493 w516 w532 w540 w557 w580 w597]
              disable-tunnel: w331 -> [w343 w349 w369 w383 w400 w425 w430 w447 w468 w485 w492 w515 w531 w539 w556 w579 w596]
              disable-tunnel: w330 -> [w342 w348 w370 w382 w401 w424 w431 w446 w469 w484 w491 w514 w530 w538 w555 w578 w595]
              disable-tunnel: w329 -> [w341 w347 w371 w381 w402 w423 w432 w445 w470 w483 w490 w513 w529 w537 w554 w577 w594]
              disable-tunnel: w328 -> [w340 w352 w373 w380 w403 w421 w433 w444 w472 w481 w488 w511 w528 w536 w551 w576 w591]
              disable-tunnel: [w339 w358 w365 w391 w412 w413 w435 w450 w465 w473 w495 w503 w519 w542 w559 w566 w590] -> w327
              disable-tunnel: [w338 w357 w364 w390 w411 w414 w436 w451 w464 w474 w496 w504 w520 w543 w560 w567 w589] -> w326
              disable-tunnel: [w337 w356 w363 w389 w410 w415 w437 w452 w463 w475 w497 w505 w521 w544 w561 w568 w588] -> w325
              disable-tunnel: [w336 w355 w362 w388 w409 w416 w438 w453 w462 w476 w498 w506 w522 w545 w562 w569 w587] -> w324
              disable-tunnel: [w335 w354 w361 w387 w408 w417 w439 w454 w461 w477 w499 w507 w523 w546 w550 w571 w586] -> w323
              disable-tunnel: [w334 w353 w372 w384 w405 w420 w440 w455 w458 w480 w500 w510 w524 w547 w563 w570 w584] -> w322
              disable-tunnel: [_ w346 w366 w386 w407 w418 w442 w457 w460 w478 w502 w508 w525 w549 w565 w572 w585] -> w321
              disable-tunnel: w320 -> [_ _ w360 w379 w404 w422 w434 w443 w471 w482 w489 w512 w527 w535 w552 w574 w592]
              disable-tunnel: [_ _ w359 w385 w406 w419 w441 w456 w459 w479 w501 w509 w526 w548 w564 w573 w582] -> w319
              disable-tunnel: w318 -> [_ _ _ _ _ _ _ _ _ _ _ _ w518 w534 w553 w575 w593]
              disable-tunnel: w317 -> [_ _ _ _ _ _ _ _ _ _ _ _ _ _ _ _ w583]
              disable-tunnel: [_ _ _ _ _ _ _ _ _ _ _ _ _ _ _ _ w582] -> w316
              frame Disabled {
                n35 = call "SubPanel_DataCollection_Rev11.vi"("DCPowerInformationClusterArray_Input"=w345, "VISAPowerInfoInputArray"=w344, "Run Data SubPanel Input"=w343, "RF Block Parameters"=w342, "Oscilloscope Info Array"=w341, "error in"=w340) -> ("DCPowerInformationClusterArray_Output"=w339:T12, "VISAPowerInfoInputOutput"=w338:T14, "Run Data SubPanel Output"=w337:T9, "RF Block Parameters Output"=w336:T3, "Oscilloscope Info Array Output"=w335:T17, "error out"=w334:errorcluster)  [unwired: 16 in]
              }
              frame Disabled {
                n36 = call "SubPanel_DataCollection_Rev11_v2.vi"("DCPowerInformationClusterArray_Input"=w351, "VISAPowerInfoInputArray"=w350, "Run Data SubPanel Input"=w349, "RF Block Parameters"=w348, "Oscilloscope Info Array"=w347, "error in"=w352) -> ("DCPowerInformationClusterArray_Output"=w358:T12, "VISAPowerInfoInputOutput"=w357:T14, "Run Data SubPanel Output"=w356:T9, "RF Block Parameters Output"=w355:T3, "Oscilloscope Info Array Output"=w354:T17, "Reinitialize?"=w346:bool, "error out"=w353:errorcluster)  [unwired: 15 in]
              }
              frame Disabled {
                n37 = call "SubPanel_DataCollection_Rev11_v3.vi"("DCPowerInformationClusterArray_Input"=w367, "VISAPowerInfoInputArray"=w368, "Run Data SubPanel Input"=w369, "RF Block Parameters"=w370, "Oscilloscope Info Array"=w371, "New Run?"=w360, "error in"=w373) -> ("DCPowerInformationClusterArray_Output"=w365:T12, "VISAPowerInfoInputOutput"=w364:T14, "Run Data SubPanel Output"=w363:T9, "RF Block Parameters Output"=w362:T3, "Oscilloscope Info Array Output"=w361:T17, "Reinitialize?"=w366:bool, "Data Was Collected?"=w359:bool, "error out"=w372:errorcluster)  [unwired: 13 in]
              }
              frame Disabled {
                n38 = call "SubPanel_DataCollection_Rev11_v4.vi"("DCPowerInformationClusterArray_Input"=w393, "VISAPowerInfoInputArray"=w392, "Run Data SubPanel Input"=w383, "RF Block Parameters"=w382, "Oscilloscope Info Array"=w381, "New Run?"=w379, "error in"=w380) -> ("data iterating in loop"=w374:T19, "each channel cluster"=w375:T19, "Array of all channels?"=w378:dbl[][], "all channel clusters as a large array"=w376:T20, "data going into the binary file"=w377:T21, "DCPowerInformationClusterArray_Output"=w391:T12, "VISAPowerInfoInputOutput"=w390:T14, "Run Data SubPanel Output"=w389:T9, "RF Block Parameters Output"=w388:T3, "Oscilloscope Info Array Output"=w387:T17, "Reinitialize?"=w386:bool, "Data Was Collected?"=w385:bool, "error out"=w384:errorcluster)  [unwired: 8 in]
              }
              frame Disabled {
                n39 = call "SubPanel_DataCollection_Rev11_v5.vi"("DCPowerInformationClusterArray_Input"=w398, "VISAPowerInfoInputArray"=w399, "Run Data SubPanel Input"=w400, "RF Block Parameters"=w401, "Oscilloscope Info Array"=w402, "New Run?"=w404, "error in"=w403) -> ("data iterating in loop"=w395:T19, "each channel cluster"=w396:T19, "Array of all channels?"=w394:dbl[][], "all channel clusters as a large array"=w397:T20, "DCPowerInformationClusterArray_Output"=w412:T12, "VISAPowerInfoInputOutput"=w411:T14, "Run Data SubPanel Output"=w410:T9, "RF Block Parameters Output"=w409:T3, "Oscilloscope Info Array Output"=w408:T17, "Reinitialize?"=w407:bool, "Data Was Collected?"=w406:bool, "error out"=w405:errorcluster)  [unwired: 8 in, 1 out]
              }
              frame Disabled {
                n40 = call "SubPanel_DataCollection_Rev11_v6.vi"("DCPowerInformationClusterArray_Input"=w427, "VISAPowerInfoInputArray"=w426, "Run Data SubPanel Input"=w425, "RF Block Parameters"=w424, "Oscilloscope Info Array"=w423, "New Run?"=w422, "error in"=w421) -> ("DCPowerInformationClusterArray_Output"=w413:T12, "VISAPowerInfoInputOutput"=w414:T14, "Run Data SubPanel Output"=w415:T9, "RF Block Parameters Output"=w416:T3, "Oscilloscope Info Array Output"=w417:T17, "Reinitialize?"=w418:bool, "Data Was Collected?"=w419:bool, "error out"=w420:errorcluster)  [unwired: 13 in]
              }
              frame Disabled {
                n41 = call "SubPanel_DataCollection_Rev11_v7.vi"("DCPowerInformationClusterArray_Input"=w428, "VISAPowerInfoInputArray"=w429, "Run Data SubPanel Input"=w430, "RF Block Parameters"=w431, "Oscilloscope Info Array"=w432, "New Run?"=w434, "error in"=w433) -> ("DCPowerInformationClusterArray_Output"=w435:T12, "VISAPowerInfoInputOutput"=w436:T14, "Run Data SubPanel Output"=w437:T9, "RF Block Parameters Output"=w438:T3, "Oscilloscope Info Array Output"=w439:T17, "Reinitialize?"=w442:bool, "Data Was Collected?"=w441:bool, "error out"=w440:errorcluster)  [unwired: 12 in, 1 out]
              }
              frame Disabled {
                n42 = call "SubPanel_DataCollection_Rev11_v8.vi"("DCPowerInformationClusterArray_Input"=w449, "VISAPowerInfoInputArray"=w448, "Run Data SubPanel Input"=w447, "RF Block Parameters"=w446, "Oscilloscope Info Array"=w445, "New Run?"=w443, "error in"=w444) -> ("DCPowerInformationClusterArray_Output"=w450:T12, "VISAPowerInfoInputOutput"=w451:T14, "Run Data SubPanel Output"=w452:T9, "RF Block Parameters Output"=w453:T3, "Oscilloscope Info Array Output"=w454:T17, "Reinitialize?"=w457:bool, "Data Was Collected?"=w456:bool, "error out"=w455:errorcluster)  [unwired: 12 in, 1 out]
              }
              frame Disabled {
                n43 = call "SubPanel_DataCollection_Rev11_v9.vi"("DCPowerInformationClusterArray_Input"=w466, "VISAPowerInfoInputArray"=w467, "Run Data SubPanel Input"=w468, "RF Block Parameters"=w469, "Oscilloscope Info Array"=w470, "New Run?"=w471, "error in"=w472) -> ("DCPowerInformationClusterArray_Output"=w465:T12, "VISAPowerInfoInputOutput"=w464:T14, "Run Data SubPanel Output"=w463:T9, "RF Block Parameters Output"=w462:T3, "Oscilloscope Info Array Output"=w461:T17, "Reinitialize?"=w460:bool, "Data Was Collected?"=w459:bool, "error out"=w458:errorcluster)  [unwired: 13 in]
              }
              frame Disabled {
                n44 = call "SubPanel_DataCollection_Rev11_v10.vi"("DCPowerInformationClusterArray_Input"=w487, "VISAPowerInfoInputArray"=w486, "Run Data SubPanel Input"=w485, "RF Block Parameters"=w484, "Oscilloscope Info Array"=w483, "New Run?"=w482, "error in"=w481) -> ("DCPowerInformationClusterArray_Output"=w473:T12, "VISAPowerInfoInputOutput"=w474:T14, "Run Data SubPanel Output"=w475:T9, "RF Block Parameters Output"=w476:T3, "Oscilloscope Info Array Output"=w477:T17, "Reinitialize?"=w478:bool, "Data Was Collected?"=w479:bool, "error out"=w480:errorcluster)  [unwired: 13 in]
              }
              frame Disabled {
                n45 = call "SubPanel_DataCollection_Rev11_v11.vi"("DCPowerInformationClusterArray_Input"=w494, "VISAPowerInfoInputArray"=w493, "Run Data SubPanel Input"=w492, 3:w491, "Oscilloscope Info Array"=w490, "New Run?"=w489, "error in"=w488) -> ("DCPowerInformationClusterArray_Output"=w495:T12, "VISAPowerInfoInputOutput"=w496:T14, "Run Data SubPanel Output"=w497:T9, "RF Block Parameters Output"=w498:T3, "Oscilloscope Info Array Output"=w499:T17, "Reinitialize?"=w502:bool, "Data Was Collected?"=w501:bool, "error out"=w500:errorcluster)  [unwired: 13 in]
              }
              frame Disabled {
                n46 = call "SubPanel_DataCollection_Rev11_v12.vi"("DCPowerInformationClusterArray_Input"=w517, "VISAPowerInfoInputArray"=w516, "Run Data SubPanel Input"=w515, "RF Block Input Array"=w514, "Oscilloscope Info Array"=w513, "New Run?"=w512, "error in"=w511) -> ("DCPowerInformationClusterArray_Output"=w503:T12, "VISAPowerInfoInputOutput"=w504:T14, "Run Data SubPanel Output"=w505:T9, "RF Subpanel Output"=w506:T3[], "Oscilloscope Info Array Output"=w507:T17, "Reinitialize?"=w508:bool, "Data Was Collected?"=w509:bool, "error out"=w510:errorcluster)  [unwired: 13 in]
              }
              frame Disabled {
                n47 = call "SubPanel_DataCollection_Rev11_v13.vi"("DCPowerInformationClusterArray_Input"=w533, "VISAPowerInfoInputArray"=w532, "Run Data SubPanel Input"=w531, "RF Block Input Array"=w530, "Oscilloscope Info Array"=w529, "Plot Color Array"=w518, "New Run?"=w527, "error in"=w528) -> ("DCPowerInformationClusterArray_Output"=w519:T12, "VISAPowerInfoInputOutput"=w520:T14, "Run Data SubPanel Output"=w521:T9, "RF Subpanel Output"=w522:T3[], "Oscilloscope Info Array Output"=w523:T17, "Reinitialize?"=w525:bool, "Data Was Collected?"=w526:bool, "error out"=w524:errorcluster)  [unwired: 12 in]
              }
              frame Disabled {
                n48 = call "SubPanel_DataCollection_Rev11_v14.vi"("DCPowerInformationClusterArray_Input"=w541, "VISAPowerInfoInputArray"=w540, "Run Data SubPanel Input"=w539, "RF Block Input Array"=w538, "Oscilloscope Info Array"=w537, "Plot Color Array"=w534, "New Run?"=w535, "error in"=w536) -> ("DCPowerInformationClusterArray_Output"=w542:T12, "VISAPowerInfoInputOutput"=w543:T14, "Run Data SubPanel Output"=w544:T9, "RF Subpanel Output"=w545:T3[], "Oscilloscope Info Array Output"=w546:T17, "Reinitialize?"=w549:bool, "Data Was Collected?"=w548:bool, "error out"=w547:errorcluster)  [unwired: 12 in]
              }
              frame Disabled {
                n49 = call "SubPanel_DataCollection_Rev11_v15.vi"("DCPowerInformationClusterArray_Input"=w558, "VISAPowerInfoInputArray"=w557, "Run Data SubPanel Input"=w556, "RF Block Input Array"=w555, "Oscilloscope Info Array"=w554, "Plot Color Array"=w553, "New Run?"=w552, "error in"=w551) -> ("DCPowerInformationClusterArray_Output"=w559:T12, "VISAPowerInfoInputOutput"=w560:T14, "Run Data SubPanel Output"=w561:T9, "RF Subpanel Output"=w562:T3[], "Oscilloscope Info Array"=w550:T8, "Reinitialize?"=w565:bool, "Data Was Collected?"=w564:bool, "error out"=w563:errorcluster)  [unwired: 12 in]
              }
              frame Disabled {
                n50 = call "SubPanel_DataCollection_Rev11_v16.vi"("DCPowerInformationClusterArray_Input"=w581, "VISAPowerInfoInputArray"=w580, "Run Data SubPanel Input"=w579, "RF Block Input Array"=w578, "Oscilloscope Info Array"=w577, "Plot Color Array"=w575, "New Run?"=w574, "error in"=w576) -> ("DCPowerInformationClusterArray_Output"=w566:T15, "VISAPowerInfoInputOutput"=w567:T14, "Run Data SubPanel Output"=w568:T9, "RF Subpanel Output"=w569:T3[], "Oscilloscope Info Array"=w571:T8, "Reinitialize?"=w572:bool, "Data Was Collected?"=w573:bool, "error out"=w570:errorcluster)  [unwired: 12 in]
              }
              frame Enabled {
                n51 = case shown="\"Single Event Latchup\", Default" w583 {
                  tunnel: w598 -> [w614 w621]
                  tunnel: w597 -> [w613 w620]
                  tunnel: w596 -> [w612 w617]
                  tunnel: w595 -> [w611 w615]
                  tunnel: w594 -> [w610 w616]
                  tunnel: w593 -> [w609 _]
                  tunnel: w592 -> [w608 _]
                  tunnel: w591 -> [w607 w623]
                  tunnel: [w606 w621] -> w590
                  tunnel: [w605 w620] -> w589
                  tunnel: [w604 w617] -> w588
                  tunnel: [w603 w615] -> w587
                  tunnel: [w602 w616] -> w586
                  tunnel: [w601 FALSE ("Reinitialize?")] -> w585
                  tunnel: [w600 TRUE ("Data Was Collected?")] -> w582
                  tunnel: [w599 w622] -> w584
                  frame "Single Event Latchup", Default {
                    n52 = call "SubPanel_DataCollection_Rev11_v17.vi"("DCPowerInformationClusterArray_Input"=w614, "VISAPowerInfoInputArray"=w613, "Run Data SubPanel Input"=w612, "RF Block Input Array"=w611, "Oscilloscope Configuration Input Array"=w610, "Plot Color Array"=w609, "New Run?"=w608, "error in"=w607) -> ("DCPowerInformationClusterArray_Output"=w606:T1[], "VISAPowerInfoOutputArray"=w605:T2[], "Run Data SubPanel Output"=w604:T9, "RF Subpanel Output"=w603:T3[], "Oscilloscope Info Array"=w602:T8, "Reinitialize?"=w601:bool, "Data Was Collected?"=w600:bool, "error out"=w599:errorcluster)  [unwired: 12 in]
                  }
                  frame "Single Event Transient" {
                    n53 = call "StandAlone_TransientDataCollection_Overhaul.vi"("error in"=w623, "Oscilloscope Configuration Array"=w616) -> ("error out"=w622:errorcluster)  [unwired: 9 in]
                  }
                }
              }
            }
          }
          frame #1 {
            n54 = case shown="True" w636 {
              tunnel: [bool[] [TRUE, TRUE, TRUE, TRUE] bool[] [FALSE, FALSE, FALSE, FALSE]] -> w638
              tunnel: ["DataCollection_Block" "Initialize"] -> w637
              tunnel: w634 -> [_ w657]
              tunnel: w632 -> [w640 w656]
              tunnel: w633 -> [w641 w655]
              tunnel: w628 -> [w642 w654]
              tunnel: w627 -> [w643 w653]
              tunnel: w625 -> [w644 w652]
              tunnel: [w640 w651] -> w631
              tunnel: [w641 w650] -> w630
              tunnel: [w642 w649] -> w629
              tunnel: [w643 w648] -> w626
              tunnel: [w644 w647] -> w624
              frame False {
              }
              frame True {
                n55 = case shown="True" w657 {
                  tunnel: w656 -> [w662 w672]
                  tunnel: w655 -> [w660 w671]
                  tunnel: w654 -> [w661 w670]
                  tunnel: w653 -> [w663 w673]
                  tunnel: w652 -> [w664 w674]
                  tunnel: [w662 w669] -> w651
                  tunnel: [w660 w668] -> w650
                  tunnel: [w661 w667] -> w649
                  tunnel: [w663 w666] -> w648
                  tunnel: [w664 w665] -> w647
                  frame False {
                  }
                  frame True {
                    n56 = call "Closing_Sessions.vi"("DCPowerInformationClusterArray_Input"=w672, "Oscilloscope Configuration Input Array"=w673, "error in (no error)"=w674, "RF Block Input Array"=w670, "VISAPowerInfoInputArray"=w671) -> ("Oscilloscope Configuration Output Array"=w666:T8, "DCPowerInformationClusterArray_Output"=w669:T22, "error out"=w665:errorcluster, "VISAPowerInfo Output Array"=w668:T2[], "RF Block Output Array"=w667:T3[])
                  }
                }
              }
            }
          }
        }
      }
      frame "Initialize", Default {
        # "Forces you to always set up where you want to put the data first"
        # "This checks if you have completed all of the instrument configuration pages. You will not be able to begin data collection if you don't"
        n57 = case shown="True" w675 {
          tunnel: w676 -> [w694 w759]
          tunnel: [w693 w759] -> w686
          tunnel: w685 -> [w692 _]
          tunnel: [w690 w761] -> w684
          frame False {
            n58 = case shown="True" "Reset" {
              tunnel: w694 -> [w755 _]
              tunnel: [w755 bool[] [FALSE, FALSE, FALSE, FALSE]] -> w693
              tunnel: [w753 w756] -> w701
              tunnel: w692 -> [w753 w756]
              frame False {
                n59 = Wait (ms)(milliseconds to wait=u32 50) -> ()  [unwired: 1 out]
              }
              frame True {
              }
            }
            n60 = Build Array("Data Block", "Power Block", "RF Block", "Oscilloscope Block", "Data Collection Block") -> (w700:bool[])
            n61 = for {
              tunnel: w700 -> [w749] mode=indexing
              shift-right: [w748] -> w689
              shift-left: 0 -> [w747]
              tunnel: [w745] -> w691
              tunnel: w701 -> [w745]
              i -> [w750]
              n62 = Increment(x=w750) -> (x+1=w746:i32)
              n63 = case shown="True" w749 {
                tunnel: [w751 w752] -> w748
                tunnel: w747 -> [w751 _]
                tunnel: w746 -> [_ w752]
                frame False {
                }
                frame True {
                }
              }
            }
            n64 = case shown="3" w689 {
              tunnel: [w702 "Data_Block_DECISION" w708 w715 w725 w733] -> w690
              tunnel: w691 -> [w702 _ _ _ _ _]
              tunnel: w693 -> [_ _ w705 w712 w724 w731]
              frame 0, Default {
                n65 = flat-sequence {
                  frame #0 {
                    n66 = Wait (ms)(milliseconds to wait=u32 50) -> ()  [unwired: 1 out]
                  }
                  frame #1 {
                  }
                }
              }
              frame 1 {
              }
              frame 3 {
                n67 = Index Array(array=w705, index=0) -> (element=w706:bool)
                n68 = case shown="False" w706 {
                  tunnel: ["Data_Block_DECISION" "RF_Block"] -> w708
                  frame False {
                    n69 = call "Display Message to User"("Message"="Please Configure the DUT information before continuing") -> ()  [unwired: 9 in, 2 out]
                  }
                  frame True {
                  }
                }
              }
              frame 2 {
                n70 = Index Array(array=w712, index=0) -> (element=w713:bool)
                n71 = case shown="False" w713 {
                  tunnel: [w716 "Power_Block"] -> w715
                  frame False {
                    n72 = Two Button Dialog(message="Please Configure the DUT information before continuing", 1:"Ok" ("F button name (\"Cancel\")"), 2:"I'm going in anyway" ("T button name (\"OK\")")) -> (T button?=w717:bool)
                    n73 = case shown="False" w717 {
                      tunnel: ["Data_Block_DECISION" "Power_Block"] -> w716
                      frame False {
                        (unwired) "Data_Block"
                      }
                      frame True {
                      }
                    }
                  }
                  frame True {
                  }
                }
              }
              frame 4 {
                n74 = Index Array(array=w724, index=0) -> (element=w726:bool)
                n75 = case shown="False" w726 {
                  tunnel: ["Data_Block_DECISION" "Oscilloscope_Block"] -> w725
                  frame False {
                    n76 = call "Display Message to User3"("Message"="Please Configure the DUT information before continuing") -> ()  [unwired: 9 in, 2 out]
                  }
                  frame True {
                  }
                }
              }
              frame 5 {
                n77 = disable-structure shown="Disabled" {
                  disable-tunnel: [w735 w740] -> w732
                  disable-tunnel: w731 -> [w734 w741]
                  frame Disabled {
                    n78 = for {
                      tunnel: w734 -> [w739] mode=indexing
                      shift-right: [w737] -> w735
                      shift-left: TRUE ("y") -> [w738]
                      n79 = And(x=w739, y=w738) -> (x .and. y?=w737:bool)
                    }
                  }
                  frame Enabled {
                    n80 = And Array Elements(Boolean array=w741) -> (logical AND=w740:bool)
                  }
                }
                n81 = case shown="False" w732 {
                  tunnel: ["Initialize" "DataCollection_Block"] -> w733
                  frame False {
                    n82 = call "Display Message to User4"("Message"="Ensure you have configured everything") -> ()  [unwired: 9 in, 2 out]
                  }
                  frame True {
                  }
                }
              }
            }
          }
          frame True {
            (unwired) -1 ("x")
            n83 = for {
              tunnel: w759 -> [w774] mode=indexing
              shift-right: [w778] -> w760
              shift-left: -1 -> [w777]
              shift-right: [w775] -> _
              shift-left: TRUE -> [w771]
              i -> [w776]
              n84 = Not(x=w774) -> (.not. x?=w773:bool)
              n85 = And(x=w771, y=w773) -> (x .and. y?=w772:bool)
              n86 = case shown="False" w772 {
                tunnel: [w779 w782] -> w778
                tunnel: w777 -> [w779 _]
                tunnel: w776 -> [_ w782]
                tunnel: [w780 FALSE] -> w775
                tunnel: w771 -> [w780 _]
                frame False {
                }
                frame True {
                }
              }
            }
            n87 = And Array Elements(Boolean array=w759) -> (logical AND=w758:bool)
            n88 = case shown="False" w758 {
              tunnel: [w764 "DataCollection_Block"] -> w761
              tunnel: w760 -> [w765 _]
              frame False {
                n89 = case shown="2" w765 {
                  tunnel: [" Data_Block " "Power_Block" "RF_Block" "Oscilloscope_Block"] -> w764
                  frame 0, Default {
                    n90 = call "Display Message to User2"() -> ()  [unwired: 10 in, 2 out]
                  }
                  frame 1 {
                  }
                  frame 2 {
                  }
                  frame 3 {
                    # "Oscilloscope_Block"
                  }
                }
              }
              frame True {
              }
            }
          }
        }
      }
      frame "Data_Block_DECISION" {
        n91 = Bundle("DCPowerInformationClusterArray_Input"=w800, "VISAPowerInfoInputArray"=w799, "RF Block Input Array"=w798, "Oscilloscope Configuration Input Array"=w797) -> (w790:T6)  [unwired: 1 in]
        n92 = disable-structure shown="Enabled" {
          disable-tunnel: [w808 w811] -> w801
          disable-tunnel: w792 -> [w807 w813]
          disable-tunnel: [w806 w812] -> w791
          disable-tunnel: w790 -> [w805 w815]
          disable-tunnel: w789 -> [w804 w814]
          disable-tunnel: [w803 w816] -> w787
          disable-tunnel: w784 -> [_ w810]
          disable-tunnel: [_ w809] -> w783
          frame Disabled {
            n93 = call "AUTO_V_MANUAL_CONFIGURATION.vi"("error in"=w807, "input path"=w804, "config file inputs"=w805) -> ("error out"=w806:errorcluster, "JSON CONFIGURED?"=w803:bool, "Instrument Configuration Clusters"=w808:T23)
          }
          frame Enabled {
            n94 = call "AUTO_V_MANUAL_CONFIGURATION.vi"("error in"=w813, "input path"=w814, "Run Data SubPanel Input"=w810, "config file inputs"=w815) -> ("error out"=w812:errorcluster, "JSON CONFIGURED?"=w816:bool, "Run Data Output"=w809:T24, "Instrument Configuration Clusters"=w811:T25)
          }
        }
        n95 = Unbundle(w801) -> ("DCPowerInformationClusterArray out"=w793:T1[], "VISAPowerInfoOutputArray"=w794:T2[], "RF Block Input Array out"=w795:T3[], "Oscilloscope Configuration Input Array"=w796:T4[])
        n96 = case shown="True" w787 {
          tunnel: ["Data_Block" "Initialize"] -> w788
          tunnel: w786 -> [w817 w821]
          tunnel: [w817 w819] -> w785
          frame False {
          }
          frame True {
            n97 = Replace Array Subset(array=w821, new element=TRUE ("new element/subarray"), index=0) -> (w819:bool[])
          }
        }
      }
    }
    "Configuration Dashboard" <- w40
    "Run Parameters" <- w36
    "RFBlockInfoArray" <- w34
    "OscilloscopeInfoArray" <- w28
    "VISAPowerOutputArray" <- w31
    "DCPowerInformationArrayOutput" <- w30
    n98 = Or(x=w20, y="stop") -> (x .or. y?=w21:bool)
  }
  n99 = call "Closing_Sessions.vi"("DCPowerInformationClusterArray_Input"=w13, "Oscilloscope Configuration Input Array"=w7, "error in (no error)"=w12, "RF Block Input Array"=w10, "VISAPowerInfoInputArray"=w11) -> ("error out"=w6:errorcluster)  [unwired: 4 out]
  "error in" <- w6
  n100 = call <vilib>:"Simple Error Handler.vi"("error in (no error)"=w6) -> ()  [unwired: 4 in, 5 out]
